vi "subvi_salvamento_dados.vi"(10 "Table":string[][](array[string]), 11 "file (use dialog)":path) -> (3 "spreadsheet string":string)   [LabVIEW 2017]
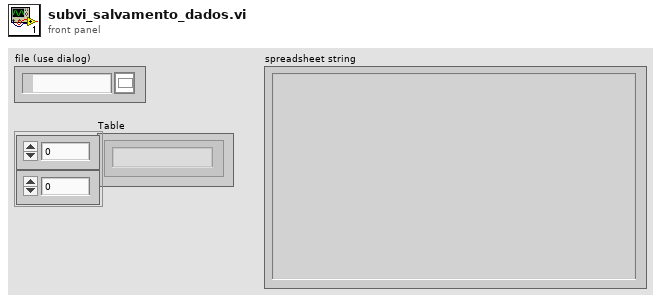
[diagram p1: front panel]
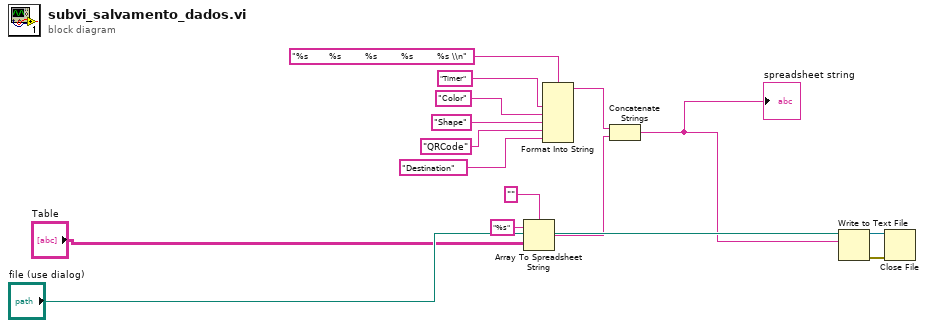
[diagram p0: block diagram]
diagram:
  n1 = Array To Spreadsheet String(delimiter (Tab)="", array="Table", 3:"%s" ("format string")) -> (spreadsheet string=w10:string)
  n2 = Format Into String(format string="%s       %s        %s        %s        %s \\n", "Timer" ("input 1"), "Color" ("input 2"), "Shape" ("input 2"), "QRCode" ("input 2"), "Destination" ("input 2")) -> (resulting string=w9:string)  [unwired: 2 in, 1 out]
  n3 = Concatenate Strings(w9, w10) -> (w12:string)
  "spreadsheet string" <- w12
  n4 = Write to Text File(file (use dialog)="file (use dialog)", text=w12) -> (refnum out=w14:refnum<file>, error out=w13:errorcluster)  [unwired: 2 in, 1 out]
  n5 = Close File(refnum=w14, error in=w13) -> ()  [unwired: 2 out]
